vi "Save_CSV.vi"(6 "Current":dbl, 8 "VSet":dbl, 9 "Vtracking":dbl format="%#_13g", 10 "Index":i32, 11 "Path":path) -> ()   [LabVIEW 2015]
uses:
  <vilib>/Utility/file.llb/Write Delimited Spreadsheet (string).vi
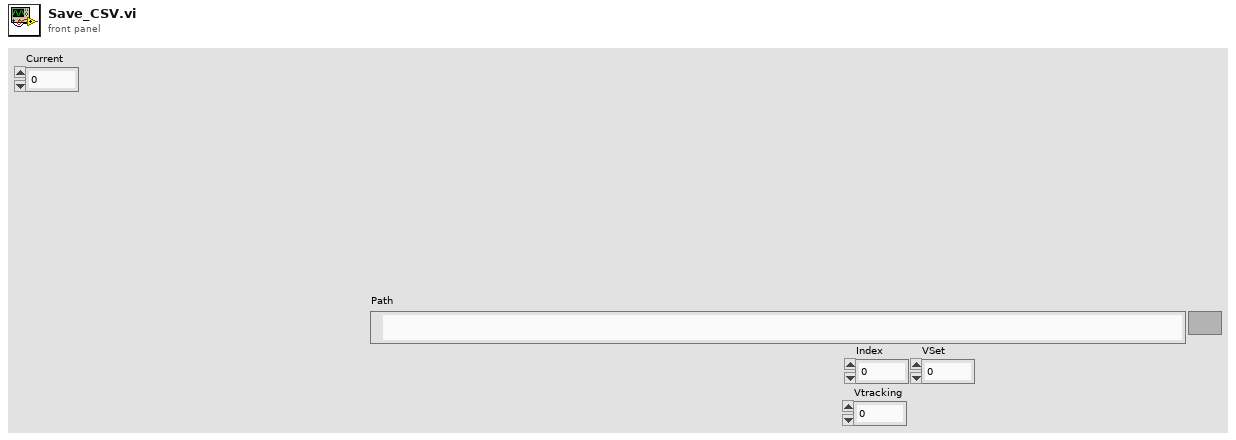
[diagram p1: front panel]
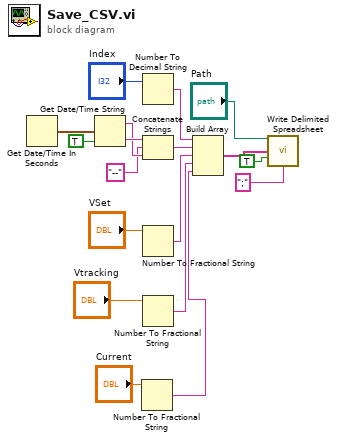
[diagram p0: block diagram]
diagram:
  n1 = Get Date/Time In Seconds() -> (seconds since 1Jan1904=w18:timestamp)
  n2 = Get Date/Time String(seconds (now)=w18, want seconds? (F)=TRUE) -> (date string=w16:string, time string=w17:string)  [unwired: 1 in]
  n3 = Number To Fractional String(number="Current") -> (F-format string=w2:string)  [unwired: 3 in]
  n4 = Number To Decimal String(number="Index") -> (decimal integer string=w6:string)  [unwired: 1 in]
  n5 = Concatenate Strings(w17, "--" ("string"), w16) -> (w14:string)
  n6 = Number To Fractional String(number="VSet") -> (F-format string=w13:string)  [unwired: 3 in]
  n7 = Number To Fractional String(number="Vtracking") -> (F-format string=w12:string)  [unwired: 3 in]
  n8 = Build Array(w6, w14, w13, w12, w2) -> (w11:string[])
  n9 = call-poly <vilib>:"Write Delimited Spreadsheet.vi"("file path (dialog if empty)"="Path", "1D data"=w11, "append to file? (F)"=TRUE, "delimiter (\\t)"=";" ("delimiter (\\t)")) -> ()  [unwired: 10 in, 2 out]
